vi "SUB subCWT.vi"(1 "f to sigma ratio":dbl=4.0 format="%#_15g", 4 "sampling rate":dbl=1.0, 5 "normalization":u16(ring) items=["Energy", "Amplitude"], 6 "user defined scales":dbl[](array[numeric]), 7 "time steps":i32=-1, 8 "error in (no error)":errorcluster, 9 "scale sampling method":u16(ring) items=["Even frequency", "Even scale"], 10 "scales":i32=128 min=1, 11 "signal":dbl[](array[numeric])) -> (0 "error out":errorcluster, 2 "scale info":variant, 3 "AWT coef":cdb[][](array[numeric]))   [LabVIEW 2017]
uses:
  <vilib>/addons/Wavelet Analysis/typedefs.llb/WA Error Code.ctl
  <vilib>/Analysis/2dsp.llb/Real FFT.vi
  <vilib>/Analysis/2dsp.llb/Inverse Complex FFT.vi
  <vilib>/addons/_Advanced Signal Processing/NI_AdvSigProcWA.lvlib
  <vilib>/Analysis/NI_AALPro.lvlib
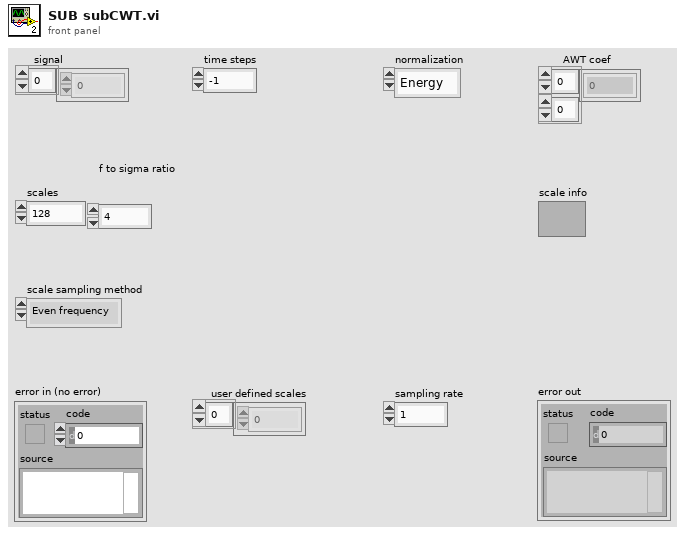
[diagram p1: front panel]
types:
  T1 = typedef "NI_AdvSigProcWA.lvlib/WA Error Code.ctl" = enum16{"No Error", "Signal Empty Error", "Invalid Selection", "Coeffs Empty Error", "Coef Level Out of Range", "Customized Color Table Error", "File Operation on RT Error", "Wavelet Type Invalid", "Invalid Scale", "Shift Value Out of Range", "Node Not On the Tree", "Filter Length <= 0", "Invalid Path", "Terminal Node", "Not Terminal  Node", "Time Step < 0", "Invalid Trend Level", "Invalid Threshold Frequency", "Optional Parameter Error", "Coeffs Dims Error", "WP Ref Error", "WFBFileFormatErr", "dt<0 Err", "RefOutOfMemErr", "Ref Invalid", "Ref Data Type Error", "Ref Index Out Of Range ", "WvltTypeWarning", "RefinementWarning", "TimeStepWarning", "InitializationWarning"}
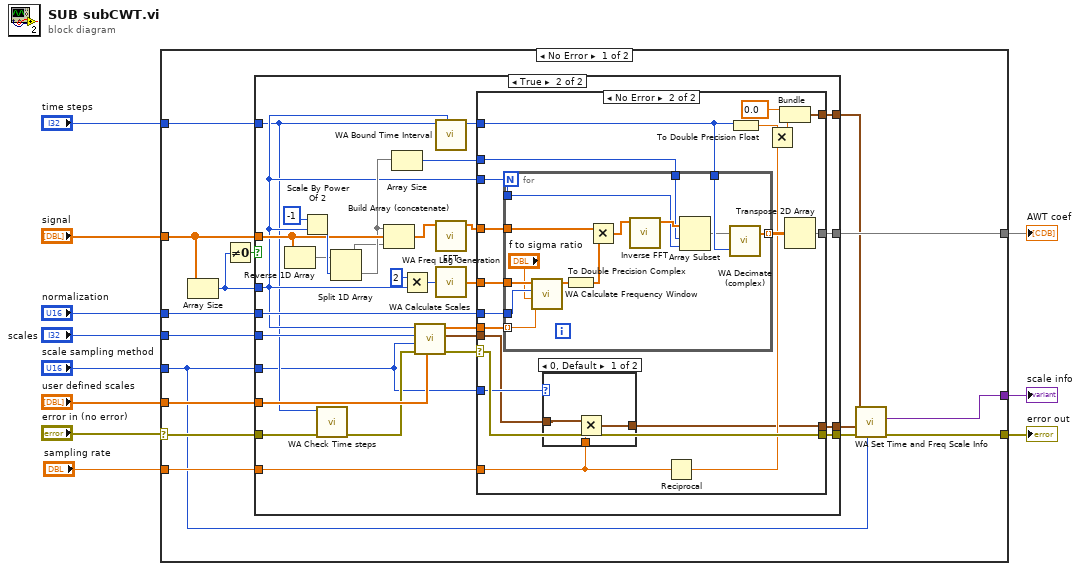
[diagram p0: block diagram]
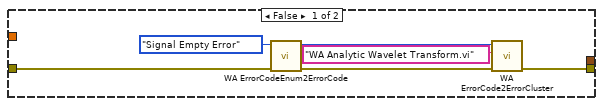
[diagram p2: hidden frame]
diagram:
  n1 = case shown="No Error" "error in (no error)" {
    selector: "error in (no error)" -> [w25 w100]
    tunnel: [w12 w100] -> w10
    tunnel: [w24 _] -> w9
    tunnel: "time steps" -> [w23 _]
    tunnel: "signal" -> [w16 _]
    tunnel: "normalization" -> [w22 _]
    tunnel: "scales" -> [w21 _]
    tunnel: "scale sampling method" -> [w14 _]
    tunnel: "user defined scales" -> [w20 _]
    tunnel: [w13 _] -> w2
    tunnel: "sampling rate" -> [w15 _]
    frame No Error {
      n2 = Array Size(array=w16) -> (size(s)=w26:i32)
      n3 = Not Equal To 0?(x=w26) -> (x != 0?=w27:bool)
      n4 = case shown="True" w27 {
        tunnel: w16 -> [_ w49]
        tunnel: w26 -> [_ w37]
        tunnel: w23 -> [_ w35]
        tunnel: w20 -> [_ w43]
        tunnel: w22 -> [_ w58]
        tunnel: [_ w57] -> w18
        tunnel: [_ w55] -> w24
        tunnel: w14 -> [_ w33]
        tunnel: w21 -> [_ w56]
        tunnel: [_ w39] -> w17
        tunnel: w25 -> [w31 w38]
        tunnel: [w30 w41] -> w19
        tunnel: w15 -> [_ w34]
        frame False {
          n5 = call <vilib>:"WA ErrorCodeEnum2ErrorCode.vi"("WA Error"=WA_Error_Code."Signal Empty Error") -> ("Error Code"=w28:i32)  [unwired: 10 out]
          n6 = call <vilib>:"WA ErrorCode2ErrorCluster.vi"("error in (no error)"=w31, "subVI name"="WA Analytic Wavelet Transform.vi", "Error Code"=w28) -> ("error out"=w30:errorcluster)  [unwired: 8 out]
        }
        frame True {
          n7 = Reverse 1D Array(array=w49) -> (reversed array=w45:dbl[])
          n8 = Scale By Power Of 2(n=-1, x=w37) -> (x*2^n=w50:i32)
          n9 = call <vilib>:"WA Check Time steps.vi"("error in (no error)"=w38, "time steps"=w35) -> ("error out"=w36:errorcluster)  [unwired: 9 out]
          n10 = Split 1D Array(array=w45, index=w50) -> (first subarray=w44:dbl[], second subarray=w48:dbl[])
          n11 = Build Array (concatenate)(w48, w49, w44) -> (w52:dbl[])
          n12 = Array Size(array=w48) -> (size(s)=w46:i32)
          n13 = Multiply(x=2, y=w37) -> (x*y=w53:i32)
          n14 = call <vilib>:"WA Calculate Scales.vi"("user defined scales"=w43, "error in (no error)"=w36, "scale sampling method"=w33, "Scales"=w56, "signal length"=w37) -> ("error out"=w42:errorcluster, "Cluster"=w40:cluster{"y":dbl, dbl}, "Scales"=w59:dbl[])  [unwired: 4 out]
          n15 = call <vilib>:"WA Bound Time Interval.vi"("signal length"=w37, "time interval"=w35) -> ("time interval out"=w47:i32)  [unwired: 1 in, 8 out]
          n16 = call-poly <vilib>:"FFT.vi"("X"=w52) -> ("FFT {X}"=w61:cdb[])  [unwired: 2 in, 8 out]
          n17 = call <vilib>:"WA Freq Lag Generation.vi"("# bins"=w53) -> ("frequency lag"=w60:dbl[])
          n18 = case shown="No Error" w42 {
            selector: w42 -> [w62 w70]
            tunnel: w61 -> [_ w81]
            tunnel: w60 -> [_ w80]
            tunnel: w59 -> [_ w78]
            tunnel: w58 -> [_ w77]
            tunnel: [_ w76] -> w57
            tunnel: [_ w74] -> w55
            tunnel: w37 -> [_ w73]
            tunnel: w47 -> [_ w72]
            tunnel: w46 -> [_ w71]
            tunnel: [w62 w70] -> w41
            tunnel: w40 -> [_ w65]
            tunnel: [_ w63] -> w39
            tunnel: w34 -> [_ w64]
            tunnel: w33 -> [_ w66]
            frame Error {
            }
            frame No Error {
              n19 = for {
                tunnel: w80 -> [w97]
                tunnel: w81 -> [w88]
                tunnel: w78 -> [w91] mode=indexing
                tunnel: w72 -> [w96]
                tunnel: [w95] -> w75 mode=indexing
                tunnel: w77 -> [w92]
                tunnel: w73 -> [w89]
                tunnel: w71 -> [w87]
                n20 = call <vilib>:"WA Calculate Frequency Window.vi"("scale"=w91, "f to sigma ratio"="f to sigma ratio", "normalization"=w92, "omega"=w97) -> ("freq win"=w99:dbl[])  [unwired: 7 out]
                n21 = To Double Precision Complex(1:w99) -> (0:w94:cdb[])
                n22 = Multiply(x=w88, y=w94) -> (x*y=w98:cdb[])
                n23 = call-poly <vilib>:"Inverse FFT.vi"("FFT {X}"=w98) -> ("X"=w93:cdb[])  [unwired: 1 in, 9 out]
                n24 = Array Subset(array=w93, index=w87, length=w89) -> (w90:cdb[])
                n25 = call <vilib>:"WA Decimate (complex).vi"("factor"=w96, "X"=w90) -> ("Decimated X"=w95:cdb[])  [unwired: 1 out]
              }
              n26 = case shown="0, Default" w66 {
                tunnel: w65 -> [w84 w85]
                tunnel: w64 -> [w83 _]
                tunnel: [w82 w85] -> w63
                frame 0, Default {
                  n27 = Multiply(x=w84, y=w83) -> (x*y=w82:cluster{"y":dbl, dbl})
                }
                frame 1 {
                }
              }
              n28 = Reciprocal(x=w64) -> (1/x=w67:dbl)
              n29 = To Double Precision Float(number=w72) -> (double precision float=w69:dbl)
              n30 = Multiply(x=w69, y=w67) -> (x*y=w68:dbl)
              n31 = Bundle(0.0, w68) -> (w76:cluster{dbl, dbl})  [unwired: 1 out]
              n32 = Transpose 2D Array(2D array=w75) -> (transposed array=w74:cdb[][])
            }
          }
        }
      }
      n33 = call <vilib>:"WA Set Time and Freq Scale Info.vi"("scale sampling method"=w14, "error in (no error)"=w19, "frequency info"=w17, "time info"=w18) -> ("error out"=w12:errorcluster, "scale info"=w13:variant)  [unwired: 6 out]
    }
    frame Error {
    }
  }
  "error out" <- w10
  "scale info" <- w2
  "AWT coef" <- w9
